vi "Set Intensity Graph X Scale.vi"(8 "error in (no error)":errorcluster, 10 "X Scale":dbl[](array[numeric]), 11 "graph_utilities in":refnum<class "graph_utilities.lvclass">) -> (0 "error out":errorcluster, 3 "graph_utilities out":refnum<class "graph_utilities.lvclass">)   [LabVIEW 2016, in "graph_utilities.lvclass"]
uses:
  graph_utilities.lvclass
  graph_utilities.lvclass/graph_utilities.ctl
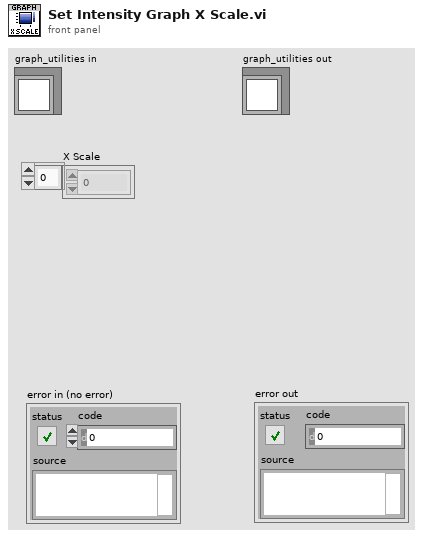
[diagram p1: front panel]
types:
  T1 = typedef "LVOffsetAndMultiplierTypeDef.ctl" = cluster{"Offset":dbl, "Multiplier":dbl}
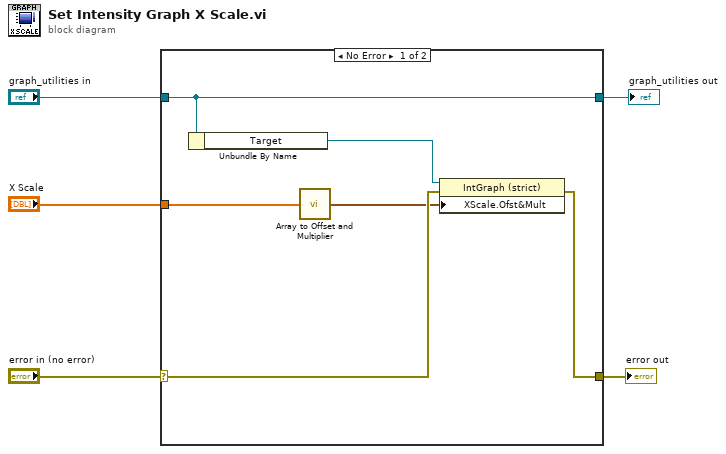
[diagram p0: block diagram]
diagram:
  n1 = case shown="No Error" "error in (no error)" {
    selector: "error in (no error)" -> [w10 w13]
    tunnel: "X Scale" -> [w9 _]
    tunnel: [w11 w13] -> w4
    tunnel: "graph_utilities in" -> [w7 w12]
    tunnel: [w7 w12] -> w1
    frame No Error {
      n2 = Unbundle By Name(w7) -> ("Target"=w6:refnum<vi>)
      n3 = call "Array to Offset and Multiplier.vi"("Array"=w9) -> ("Offset and Multiplier"=w8:T1)
      n4 = property on="Property Node" class="IntGraph (strict)"(reference=w6, error in=w10, "XScale.Ofst&Mult"=w8) -> (error out=w11:errorcluster)  [unwired: 1 out]
    }
    frame Error {
    }
  }
  "error out" <- w4
  "graph_utilities out" <- w1
